vi "PH_SRDG645.set Status.vi"(0 "i ref in":refnum<vi>, 5 "error in":errorcluster) -> (14 "i ref out":refnum<vi>, 19 "error out":errorcluster)   [LabVIEW 2014, in "PH_SRDG645.lvlib"]
doc: "This VI sets the status: In case of a device failure it is set to failure (3), otherwise to on (2). The status is indicated and published a DIM-service."
uses:
  PH_SRDG645.lvlib
  lib.lib/DimLVEvent/LVDimInterface/LVDimInterface.lvlib
  PH_StatusHandler/PH_StatusHandler.lvlib
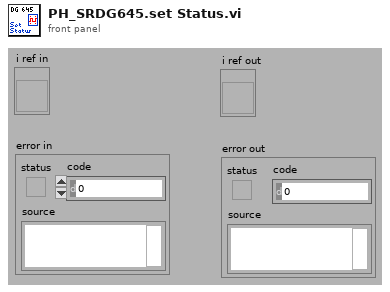
[diagram p1: front panel]
types:
  T1 = typedef "PH_StatusHandler.lvlib/PH_StatusHandler.Status.ctl" = i16
  T2 = typedef "PH_SRDG645.lvlib/PH_SRDG645.i attribute.ctl" = cluster{"GUI Refs":cluster{"Delete":refnum<vi>, "Device Errors":refnum<vi>, "Trigger":refnum<vi>, "Default Name":refnum<vi>, "Firmware Revision":refnum<vi>, "Serial Number":refnum<vi>, "Model":refnum<vi>, "Visa resource name":refnum<vi>}, "Service ID Rate":i32, "Service IDs Channelinfo":i32[], "VISA resource name":refnum<visa-resource-name>, "Device Errors":cluster{"code":i32, "Text":string}[], "Trigger":T3, "Channels":cluster{"T1":T4, "A":T4, "B":T4, "C":T4, "D":T4, "E":T4, "F":T4, "G":T4, "H":T4}, "GUI Refs Channels":refnum<vi>[], "Outputs":cluster{"AB":cluster{"Level Offset [V]":dbl, "Amplitue [V]":dbl, "Polarity":i32}, "CD":cluster{"Level Offset [V]":dbl, "Amplitue [V]":dbl, "Polarity":i32}, "EF":cluster{"Level Offset [V]":dbl, "Amplitue [V]":dbl, "Polarity":i32}, "GH":cluster{"Level Offset [V]":dbl, "Amplitue [V]":dbl, "Polarity":i32}, "T0":cluster{"Level Offset [V]":dbl, "Amplitue [V]":dbl, "Polarity":i32}}, "GUI Refs Outputs":refnum<vi>[], "Serial Number":string, "Firmweare Revision":string, "Model":string}
  T3 = typedef "PH_SRDG645.lvlib/PH_SRDG645.Trigger.ctl" = cluster{"Source":i32, "Rate [Hz]":dbl, "Level [V]":dbl}
  T4 = typedef "PH_SRDG645.lvlib/PH_SRDG645.Channel Settings.ctl" = cluster{"Delay [s]":dbl, "relative to":i32}
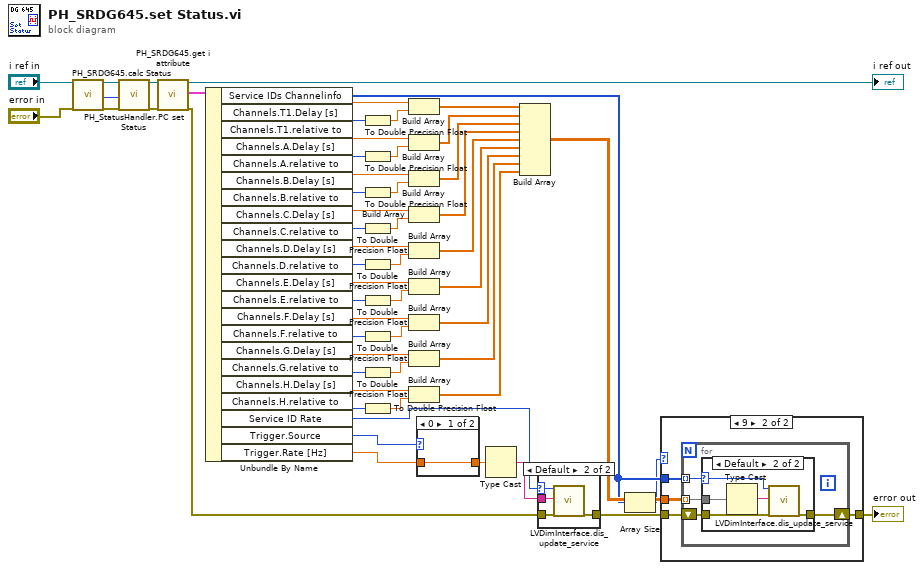
[diagram p0: block diagram]
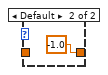
[diagram p5: hidden frame]
diagram:
  n1 = call "PH_SRDG645.calc Status.vi"("i ref in"="i ref in", "error in"="error in") -> ("i ref out"=w4:refnum<vi>, "Status"=w2:T1, "error out"=w6:errorcluster)  [unwired: 15 in]
  n2 = call "PH_StatusHandler.PC set Status.vi"("i ref in"=w4, "Status"=w2, "error in (no error)"=w6) -> ("i ref out"=w3:refnum<vi>, "error out"=w5:errorcluster)  [unwired: 15 in]
  n3 = call "PH_SRDG645.get i attribute.vi"("i ref in"=w3, "error in (no error)"=w5) -> ("i ref out"=→"i ref out":refnum<vi>, "i attribute"=w56:T2, "error out"=w1:errorcluster)  [unwired: 15 in]
  n4 = Unbundle By Name(w56) -> ("Service IDs Channelinfo"=w31:i32[], "Channels.T1.Delay [s]"=w42:dbl, "Channels.T1.relative to"=w47:i32, "Channels.A.Delay [s]"=w41:dbl, "Channels.A.relative to"=w46:i32, "Channels.B.Delay [s]"=w40:dbl, "Channels.B.relative to"=w45:i32, "Channels.C.Delay [s]"=w44:dbl, "Channels.C.relative to"=w48:i32, "Channels.D.Delay [s]"=w25:dbl, "Channels.D.relative to"=w14:i32, "Channels.E.Delay [s]"=w24:dbl, "Channels.E.relative to"=w13:i32, "Channels.F.Delay [s]"=w23:dbl, "Channels.F.relative to"=w12:i32, "Channels.G.Delay [s]"=w22:dbl, "Channels.G.relative to"=w11:i32, "Channels.H.Delay [s]"=w20:dbl, "Channels.H.relative to"=w10:i32, "Service ID Rate"=w9:i32, "Trigger.Source"=w51:i32, "Trigger.Rate [Hz]"=w52:dbl)
  n5 = To Double Precision Float(number=w47) -> (double precision float=w39:dbl)
  n6 = To Double Precision Float(number=w46) -> (double precision float=w38:dbl)
  n7 = To Double Precision Float(number=w45) -> (double precision float=w37:dbl)
  n8 = To Double Precision Float(number=w48) -> (double precision float=w43:dbl)
  n9 = To Double Precision Float(number=w14) -> (double precision float=w29:dbl)
  n10 = To Double Precision Float(number=w13) -> (double precision float=w28:dbl)
  n11 = To Double Precision Float(number=w12) -> (double precision float=w27:dbl)
  n12 = To Double Precision Float(number=w11) -> (double precision float=w26:dbl)
  n13 = To Double Precision Float(number=w10) -> (double precision float=w21:dbl)
  n14 = Build Array(w42, w39) -> (w36:dbl[])
  n15 = Build Array(w41, w38) -> (w35:dbl[])
  n16 = Build Array(w40, w37) -> (w34:dbl[])
  n17 = Build Array(w44, w43) -> (w33:dbl[])
  n18 = Build Array(w25, w29) -> (w19:dbl[])
  n19 = Build Array(w24, w28) -> (w18:dbl[])
  n20 = Build Array(w23, w27) -> (w17:dbl[])
  n21 = Build Array(w22, w26) -> (w16:dbl[])
  n22 = Build Array(w20, w21) -> (w15:dbl[])
  n23 = case shown="0" w51 {
    tunnel: w52 -> [w57 _]
    tunnel: [w57 -1.0 ("d64")] -> w53
    frame 0 {
    }
    frame Default {
    }
  }
  n24 = Type Cast(x=w53) -> (*(type *) &x=w54:string)  [unwired: 1 in]
  n25 = Build Array(w36, w35, w34, w33, w19, w18, w17, w16, w15) -> (w32:dbl[][])
  n26 = case shown="Default" w9 {
    selector: w9 -> [_ w60]
    tunnel: w1 -> [w59 w63]
    tunnel: [w59 w62] -> w49
    tunnel: w54 -> [_ w61]
    frame -1 {
    }
    frame Default {
      n27 = call "LVDimInterface.dis_update_service.vi"("my_serviceID"=w60, "data"=w61, "error in (no error)"=w63) -> ("error out"=w62:errorcluster)  [unwired: 14 in, 2 out]
    }
  }
  n28 = Array Size(array=w31) -> (size(s)=w30:i32)
  n29 = case shown="9" w30 {
    tunnel: [w64 w68] -> w50
    tunnel: w49 -> [w64 w67]
    tunnel: w32 -> [_ w66]
    tunnel: w31 -> [_ w65]
    frame Default {
    }
    frame 9 {
      n30 = for {
        shift-right: [w72] -> w68
        shift-left: w67 -> [w71]
        tunnel: w65 -> [w70] mode=indexing
        tunnel: w66 -> [w69] mode=indexing
        n31 = case shown="Default" w70 {
          selector: w70 -> [_ w74]
          tunnel: [w73 w77] -> w72
          tunnel: w71 -> [w73 w76]
          tunnel: w69 -> [_ w75]
          frame -1 {
          }
          frame Default {
            n32 = Type Cast(x=w75) -> (*(type *) &x=w78:string)  [unwired: 1 in]
            n33 = call "LVDimInterface.dis_update_service.vi"("my_serviceID"=w74, "data"=w78, "error in (no error)"=w76) -> ("error out"=w77:errorcluster)  [unwired: 14 in, 2 out]
          }
        }
      }
    }
  }
  "error out" <- w50
